vi "Status TCU Module.vi"(8 "error in (no error)":errorcluster, 11 "?":T1={"State"=enum."Idle", "Start Time"=timestamp(0 s since 1904-01-01), "Configuration"={"Cycle Period"=0.0, "Setpoint Entry"=0.0, "Output Device"=enum."Default", "Huber Ministat 230 Settings"={"VISA resource name"="", "Simulated?"=FALSE}, "Lauda Settings"={"VISA resource name"="", "Simulated?"=FALSE, "Pump Power"=2}, "Julabo FP-50 Settings"={"VISA resource name"="", "Simulated?"=FALSE, "Pump Power"=2}, "Internal Control?"=FALSE, "Huber Unistat 410 Settings"={"VISA resource name"="", "Simulated?"=FALSE}}, "Current Time"=timestamp(0 s since 1904-01-01), "First Iteration"=FALSE, "Data"={"TCU Speed"=0.0, "Temperature"=0.0}, "Process Name"="", "TCU On?"=FALSE, "Output Error"=FALSE, "Start Log"=FALSE, "Power Level Changed"=FALSE} {"Configuration"."Julabo FP-50 Settings"."Pump Power" min=0 max=8 step=1; "Configuration"."Lauda Settings"."Pump Power" min=0 max=8 step=1}) -> (0 "error out":errorcluster, 3 "State out":T1={"State"=enum."Idle", "Start Time"=timestamp(0 s since 1904-01-01), "Configuration"={"Cycle Period"=0.0, "Setpoint Entry"=0.0, "Output Device"=enum."Huber Ministat 230", "Huber Ministat 230 Settings"={"VISA resource name"="", "Simulated?"=FALSE}, "Lauda Settings"={"VISA resource name"="", "Simulated?"=FALSE, "Pump Power"=2}, "Julabo FP-50 Settings"={"VISA resource name"="", "Simulated?"=FALSE, "Pump Power"=2}, "Internal Control?"=FALSE, "Huber Unistat 410 Settings"={"VISA resource name"="", "Simulated?"=FALSE}}, "Current Time"=timestamp(0 s since 1904-01-01), "First Iteration"=FALSE, "Data"={"TCU Speed"=0.0, "Temperature"=0.0}, "Process Name"="", "TCU On?"=FALSE, "Output Error"=FALSE, "Start Log"=FALSE, "Power Level Changed"=FALSE} {"Configuration"."Julabo FP-50 Settings"."Pump Power" min=0 max=8 step=1; "Configuration"."Lauda Settings"."Pump Power" min=0 max=8 step=1})   [LabVIEW 2018, in "TCU Module.lvlib"]
uses:
  TCU Module.lvlib
  Measure Instrument/TCU State Cluster.ctl
  Measure Instrument/State Enum.ctl
  TCU Module Settings Cluster.ctl
  Measure Instrument/Output Devices.ctl
  Huber TCU/Huber Settings.ctl
  Lauda Integral XT-150 TCU/Lauda Settings.ctl
  Julabo Type 1 TCU/Julabo Type 1 TCU Folder/Julabo FP-50 Settings.ctl
  Huber Unistat 410 TCU/Huber Unistat 410 Settings.ctl
  Tag VIs/Tag FGV Operation Enum.ctl
  Shared Variables/Dynamic Shared Variables.lvlib
  Measure Instrument/TCU Module Engine.lvlib
  Huber TCU/Huber Ministat 230 TCU.lvlib
  Lauda Integral XT-150 TCU/Lauda TCU.lvlib
  Julabo Type 1 TCU/Julabo Type 1 TCU Folder/Julabo Type FP-50 TCU.lvlib
  Huber Unistat 410 TCU/Huber Unistat 410 TCU.lvlib
panel:
  # "Output Instruments"
  # "Output Instruments"
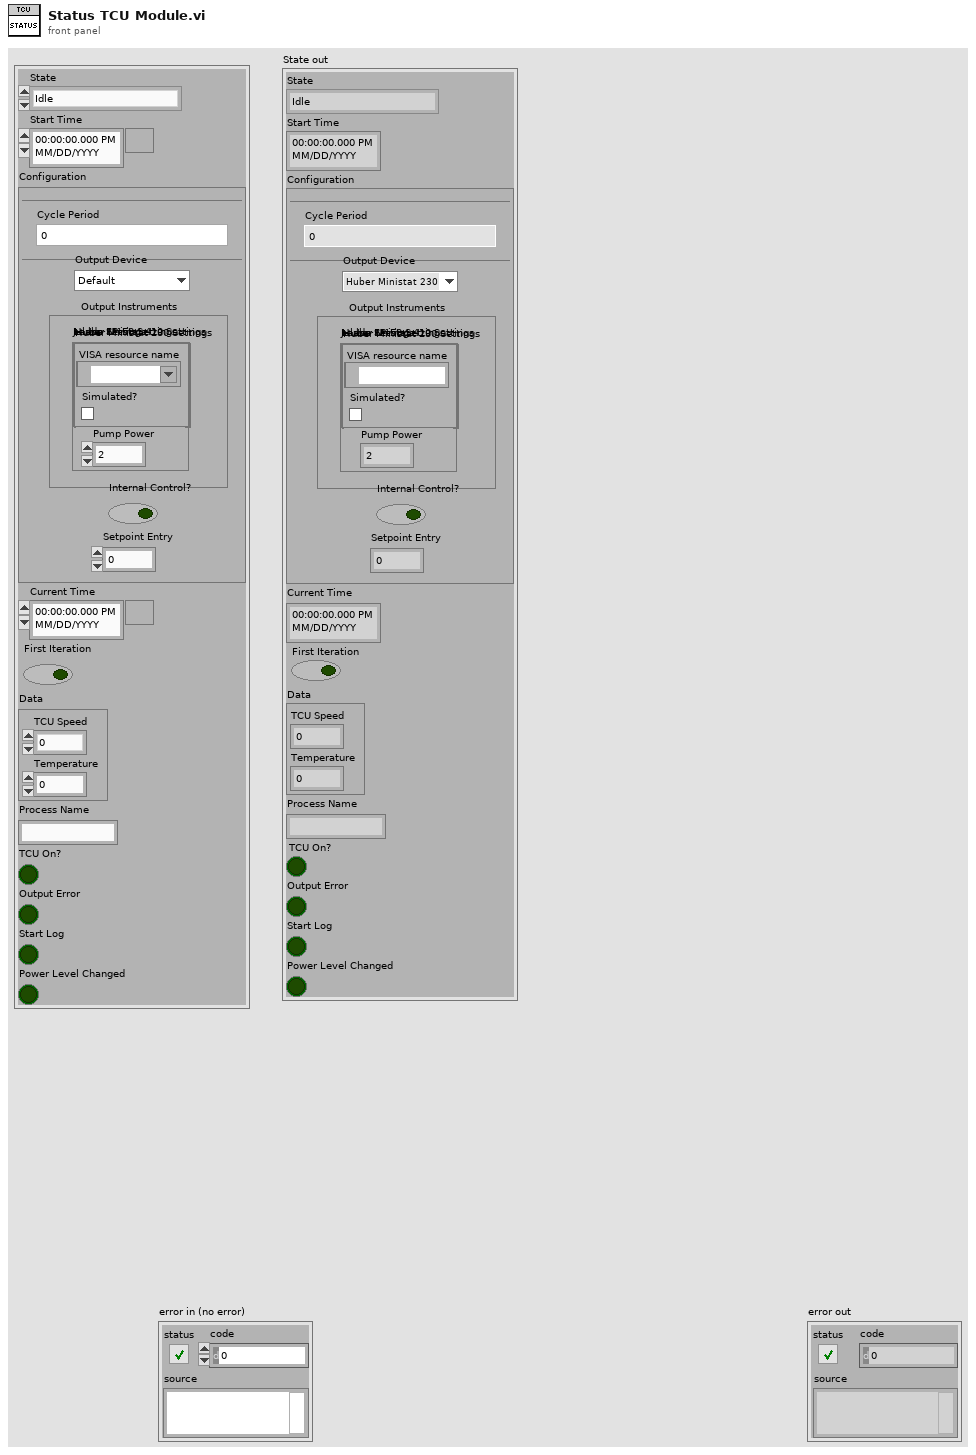
[diagram p1: front panel]
types:
  T1 = typedef "TCU Module.lvlib/TCU Module Engine.lvlib/TCU State Cluster.ctl" = cluster{"State":T2, "Start Time":timestamp, "Configuration":T3, "Current Time":timestamp, "First Iteration":bool, "Data":cluster{"TCU Speed":dbl, "Temperature":dbl}, "Process Name":string, "TCU On?":bool, "Output Error":bool, "Start Log":bool, "Power Level Changed":bool}
  T2 = typedef "TCU Module.lvlib/TCU Module Engine.lvlib/State Enum.ctl" = enum16{"Measuring", "Idle", "Paused"}
  T3 = typedef "TCU Module.lvlib/TCU Module Settings Cluster.ctl" = cluster{"Cycle Period":dbl, "Setpoint Entry":dbl, "Output Device":T4, "Huber Ministat 230 Settings":T5, "Lauda Settings":T6, "Julabo FP-50 Settings":T7, "Internal Control?":bool, "Huber Unistat 410 Settings":T8}
  T4 = typedef "Output Devices.ctl" = enum16{"Default", "Huber Ministat 230", "Huber Unistat 410", "Lauda XT-150", "Julabo FP-50"}
  T5 = typedef "Huber Ministat 230 TCU.lvlib/Huber Settings.ctl" = cluster{"VISA resource name":refnum<visa-resource-name>, "Simulated?":bool}
  T6 = typedef "Lauda TCU.lvlib/Lauda Settings.ctl" = cluster{"VISA resource name":refnum<visa-resource-name>, "Simulated?":bool, "Pump Power":i32}
  T7 = typedef "Julabo Type FP-50 TCU.lvlib/Julabo FP-50 Settings.ctl" = cluster{"VISA resource name":refnum<visa-resource-name>, "Simulated?":bool, "Pump Power":i32}
  T8 = typedef "Huber Unistat 410 TCU.lvlib/Huber Unistat 410 Settings.ctl" = cluster{"VISA resource name":refnum<visa-resource-name>, "Simulated?":bool}
  T9 = typedef "Tag FGV Operation Enum.ctl" = enum16{"Init", "Set Notification Queue", "Create Tag", "Commit", "Write Tag (Numeric)", "Write Tag (Boolean)", "Read All Tags", "Read One Tag", "Delete Tag Category", "Set Alarm Parameters (Numeric)", "Set Alarm Parameters (Boolean)", "Enable All Alarms", "Disable All Alarms", "Delete All Tags", "Read Alarms", "Ack Alarm"}
  T10 = typedef "TCU Module.lvlib/TCU Module Tag Names Cluster.ctl" = cluster{"TCU Temp":string, "Output Device Tag":string, "TCU Speed":string}
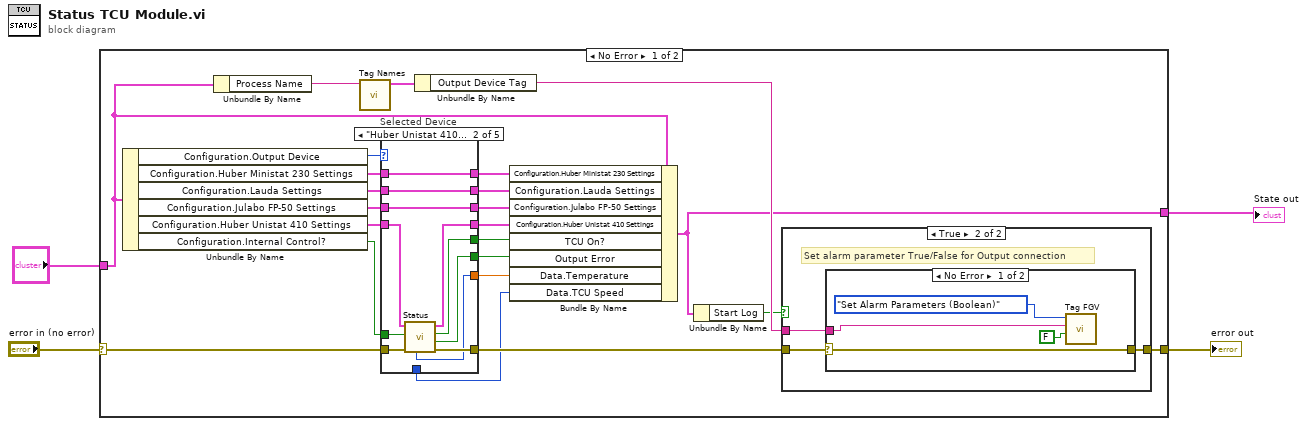
[diagram p0: block diagram]
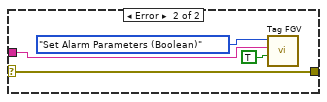
[diagram p3: hidden frame]
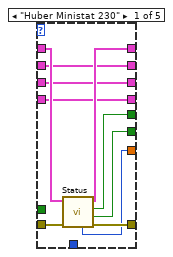
[diagram p4: hidden frame]
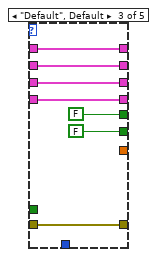
[diagram p5: hidden frame]
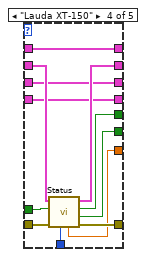
[diagram p6: hidden frame]
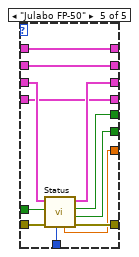
[diagram p7: hidden frame]
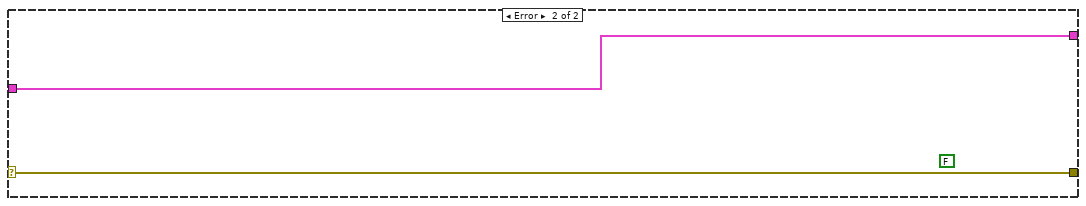
[diagram p8: hidden frame]
diagram:
  n1 = case shown="No Error" "error in (no error)" {
    selector: "error in (no error)" -> [w27 w93]
    tunnel: [w24 w93] -> w3
    tunnel: "?" -> [w19 w92]
    tunnel: [w13 w92] -> w1
    frame No Error {
      n2 = Unbundle By Name(w19) -> ("Configuration.Output Device"=w21:T4, "Configuration.Huber Ministat 230 Settings"=w20:T5, "Configuration.Lauda Settings"=w16:T6, "Configuration.Julabo FP-50 Settings"=w15:T7, "Configuration.Huber Unistat 410 Settings"=w5:T8, "Configuration.Internal Control?"=w10:bool)
      n3 = Unbundle By Name(w19) -> ("Process Name"=w22:string)
      n4 = call "Tag Names.vi"("Process Name"=w22) -> ("Pump Module Tag Names"=w23:T10)  [unwired: 8 in, 2 out]
      n5 = case "Selected Device" shown="\"Huber Unistat 410\"" w21 {
        tunnel: w20 -> [w49 w60 w64 w72 w91]
        tunnel: [w47 w53 w67 w78 w88] -> w25
        tunnel: w27 -> [w48 w52 w67 w79 w89]
        tunnel: [w46 w55 FALSE w77 w85] -> w18
        tunnel: [w45 w54 FALSE ("Connection Error") w76 w84] -> w17
        tunnel: [w44 w60 w64 w72 w91] -> w9
        tunnel: [w43 w59 w63 w75 w90] -> w8
        tunnel: w16 -> [w43 w59 w63 w74 w90]
        tunnel: [w42 w58 w62 w73 w86] -> w7
        tunnel: w15 -> [w42 w58 w62 w73 w87]
        tunnel: [w40 w50 _ w71 w83] -> w12
        tunnel: [_ _ _ w70 w82] -> w11
        tunnel: w10 -> [_ w51 _ w69 w80]
        tunnel: [w41 w56 w61 w68 w81] -> w6
        tunnel: w5 -> [w41 w57 w61 w68 w81]
        frame "Huber Ministat 230" {
          n6 = call "Status.vi"("error in (no error)"=w48, "Huber Settings"=w49) -> ("error out"=w47:errorcluster, "Connection Error"=w45:bool, "Running"=w46:bool, "Huber Settings"=w44:T5, "Temp"=w40:i32)  [unwired: 5 in]
        }
        frame "Huber Unistat 410" {
          n7 = call "Status.vi"("error in (no error)"=w52, "Internal?"=w51, "Huber Settings"=w57) -> ("error out"=w53:errorcluster, "Connection Error"=w54:bool, "Running"=w55:bool, "Huber Settings"=w56:T8, "Temperature"=w50:i32)  [unwired: 4 in]
        }
        frame "Default", Default {
        }
        frame "Lauda XT-150" {
          n8 = call "Status.vi"("error in (no error)"=w79, "Internal?"=w69, "Lauda Settings"=w74) -> ("error out"=w78:errorcluster, "Connection Error"=w76:bool, "Running"=w77:bool, "Lauda Settings"=w75:T6, "Temp"=w71:dbl, "Pump Speed"=w70:i32)  [unwired: 2 in, 1 out]
        }
        frame "Julabo FP-50" {
          n9 = call "Status.vi"("error in (no error)"=w89, "Internal?"=w80, "Julabo FP-50 Settings"=w87) -> ("error out"=w88:errorcluster, "Connection Error"=w84:bool, "Running"=w85:bool, "Julabo FP-50 Settings"=w86:T7, "Temp"=w83:dbl, "Pumpstage (out)"=w82:u8)  [unwired: 3 in]
        }
      }
      n10 = Unbundle By Name(w23) -> ("Output Device Tag"=w26:string)
      n11 = Bundle By Name(cluster=w19, "Configuration.Huber Ministat 230 Settings"=w9, "Configuration.Lauda Settings"=w8, "Configuration.Julabo FP-50 Settings"=w7, "Configuration.Huber Unistat 410 Settings"=w6, "TCU On?"=w18, "Output Error"=w17, "Data.Temperature"=w12, "Data.TCU Speed"=w11) -> (w13:T1)
      n12 = Unbundle By Name(w13) -> ("Start Log"=w14:bool)
      n13 = case shown="True" w14 {
        tunnel: w26 -> [_ w31]
        tunnel: w25 -> [w28 w30]
        tunnel: [w28 w29] -> w24
        frame False {
        }
        frame True {
          # "Set alarm parameter True/False for Output connection"
          n14 = case shown="No Error" w30 {
            selector: w30 -> [w35 w39]
            tunnel: [w35 w39] -> w29
            tunnel: w31 -> [w32 w38]
            frame No Error {
              n15 = call "Tag FGV.vi"("Data"=FALSE, "Tag Name"=w32, "Operation"=Tag_FGV_Operation_Enum."Set Alarm Parameters (Boolean)") -> ()  [unwired: 3 in, 6 out]
            }
            frame Error {
              n16 = call "Tag FGV.vi"("Data"=TRUE, "Tag Name"=w38, "Operation"=Tag_FGV_Operation_Enum."Set Alarm Parameters (Boolean)") -> ()  [unwired: 3 in, 6 out]
            }
          }
        }
      }
    }
    frame Error {
      (unwired) FALSE
    }
  }
  "error out" <- w3
  "State out" <- w1
